vi "LCR_PlotNamer.vi"(5 "Y-Axis":T1, 7 "X-Axis":T1, 11 "Graph Ref In":refnum<vi>) -> ()   [LabVIEW 2021]
uses:
  Plotting-Axis.ctl
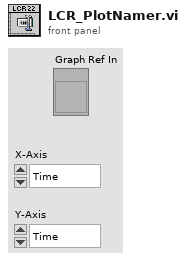
[diagram p1: front panel]
types:
  T1 = typedef "Plotting-Axis.ctl" = enum16{"Time", "Temperature", "MagneticField", "Capacitance", "Loss"}
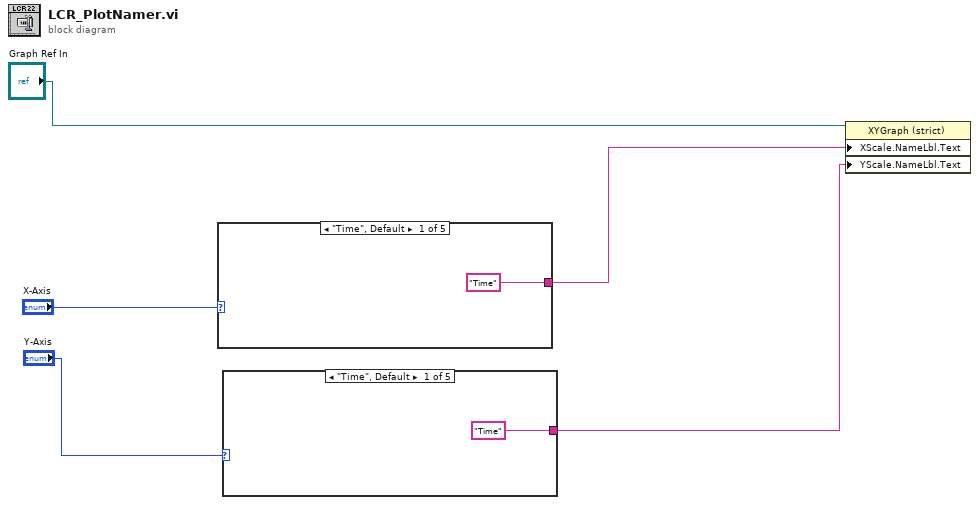
[diagram p0: block diagram]
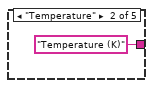
[diagram p2: hidden frame]
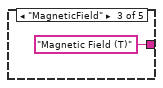
[diagram p3: hidden frame]
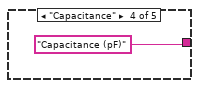
[diagram p4: hidden frame]
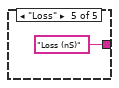
[diagram p5: hidden frame]
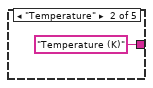
[diagram p6: hidden frame]
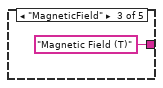
[diagram p7: hidden frame]
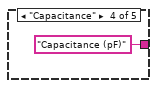
[diagram p8: hidden frame]
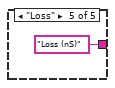
[diagram p9: hidden frame]
diagram:
  n1 = case shown="\"Time\", Default" "X-Axis" {
    tunnel: ["Time" "Temperature (K)" ("Caption.Text") "Magnetic Field (T)" ("Caption.Text") "Capacitance (pF)" ("Caption.Text") "Loss (nS)" ("Caption.Text")] -> w2
    frame "Time", Default {
    }
    frame "Temperature" {
    }
    frame "MagneticField" {
    }
    frame "Capacitance" {
    }
    frame "Loss" {
    }
  }
  n2 = case shown="\"Time\", Default" "Y-Axis" {
    tunnel: ["Time" "Temperature (K)" ("Caption.Text") "Magnetic Field (T)" ("Caption.Text") "Capacitance (pF)" ("Caption.Text") "Loss (nS)" ("Caption.Text")] -> w1
    frame "Time", Default {
    }
    frame "Temperature" {
    }
    frame "MagneticField" {
    }
    frame "Capacitance" {
    }
    frame "Loss" {
    }
  }
  n3 = property class="XYGraph (strict)"(reference="Graph Ref In", "XScale.NameLbl.Text"=w2, "YScale.NameLbl.Text"=w1) -> ()  [unwired: 1 in, 2 out]
